vi "_addProperties.vi"() -> ()   [LabVIEW 2019]
uses:
  <vilib>/JDP Science/JSONtext/JSONtext.lvlib
panel:
  in  "Property Names":string[][](array[string])
  in  "Property Values":variant[][](array[variant])
  out "<JSON> Object Out":string
  out "error out":errorcluster
  in  "error in (no error)":errorcluster
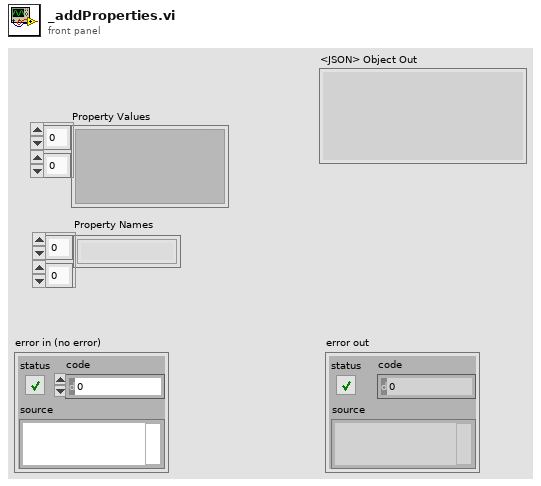
[diagram p1: front panel]
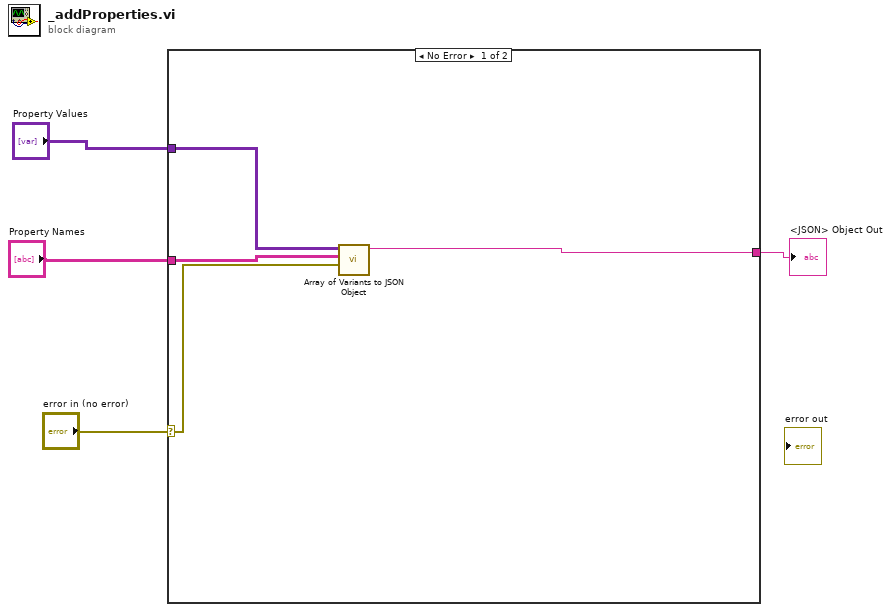
[diagram p0: block diagram]
diagram:
  n1 = case shown="No Error" "error in (no error)" {
    selector: "error in (no error)" -> [w6 _]
    tunnel: "Property Values" -> [w8 _]
    tunnel: "Property Names" -> [w7 _]
    tunnel: [w5 _] -> w3
    frame No Error {
      n2 = call <vilib>:"Array of Variants to JSON Object.vi"("error in (no error)"=w6, "Names"=w7, "Array"=w8) -> ("<JSON>"=w5:string)  [unwired: 7 in, 1 out]
    }
    frame Error {
    }
  }
  "<JSON> Object Out" <- w3
